vi "SENS_IF_FILT_STAGE_PCAT.vi"(0 "VISA IN":refnum<visa-resource-name>, 5 "error in":errorcluster, 7 "Channel":i32) -> (14 "VISA Out":refnum<visa-resource-name>, 16 "Data":string, 19 "error out":errorcluster)   [LabVIEW 2018, in "PNA-X.lvlib"]
doc: "SENSe<cnum>:IF:FILTer:STAGE3:PCATalog? \n(Read-only) Returns a list of the available parameters for the currently selected filter type. \nCritical Note \nParameters \n<cnum> Existing channel number. If unspecified, <cnum> is set to 1. \nExamples SENS:IF:FILT:STAGe3:PCAT? \nsense2:if:filter:stage3:pcatalog? \nReturn Type String \nDefault Not Applicable"
uses:
  PNA-X.lvlib
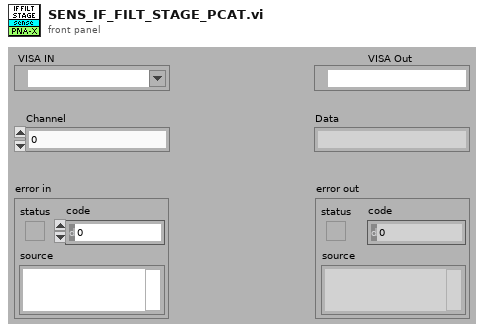
[diagram p1: front panel]
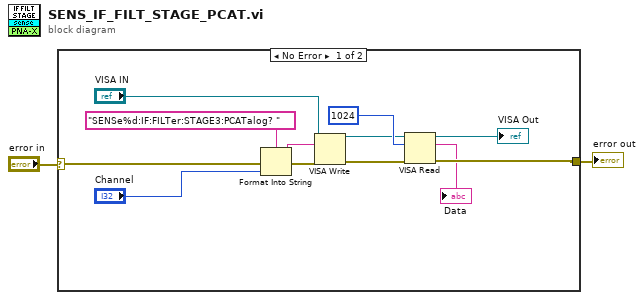
[diagram p0: block diagram]
diagram:
  n1 = case shown="No Error" "error in" {
    selector: "error in" -> [w14 w15]
    tunnel: [w5 w15] -> w1
    frame No Error {
      n2 = Format Into String(format string="SENSe%d:IF:FILTer:STAGE3:PCATalog? " ("Cmdline"), error in=w14, "Channel") -> (resulting string=w12:string, error out=w13:errorcluster)  [unwired: 1 in]
      n3 = VISA Write(VISA resource name="VISA IN", write buffer=w12, error in (no error)=w13) -> (VISA resource name out=w7:refnum<visa-resource-name>, error out=w9:errorcluster)  [unwired: 1 out]
      n4 = VISA Read(VISA resource name=w7, byte count=1024, error in (no error)=w9) -> (VISA resource name out=→"VISA Out":refnum<visa-resource-name>, read buffer=→"Data":string, error out=w5:errorcluster)  [unwired: 1 out]
    }
    frame Error {
    }
  }
  "error out" <- w1
